vi "copy.vi"(8 "error in (no error)":errorcluster, 10 "ScriptEventForCopy":refnum<class "ScriptEvent.lvclass">, 11 "SingleToneRamp in":refnum<class "SingleToneRamp.lvclass">) -> (0 "error out":errorcluster, 3 "SingleToneRamp Copy":refnum<class "SingleToneRamp.lvclass">)   [LabVIEW 2011, in "Tools.lvlib" / "Scripting.lvlib" / "SingleToneRamp.lvclass"]
uses:
  SingleToneRamp.lvclass
  ScriptEvent.lvclass
  SingleTone.lvclass
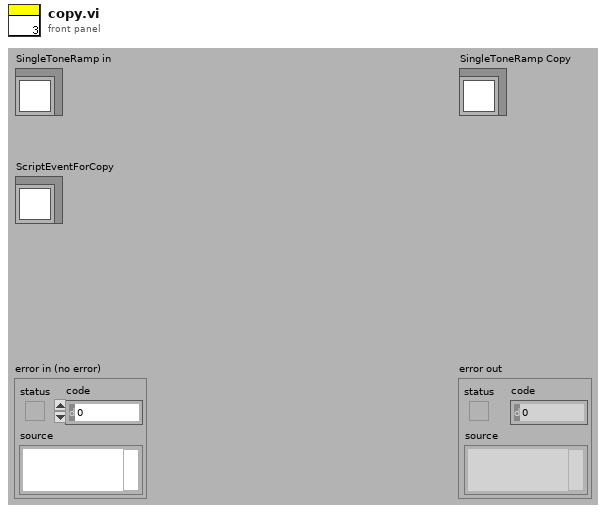
[diagram p1: front panel]
types:
  T1 = enum16{"changeValue", "pulse", "clock", "rampUp", "rampDown", "singleTone", "singleToneRamp", "playFile", "rf", "rfRamp", "delay"}
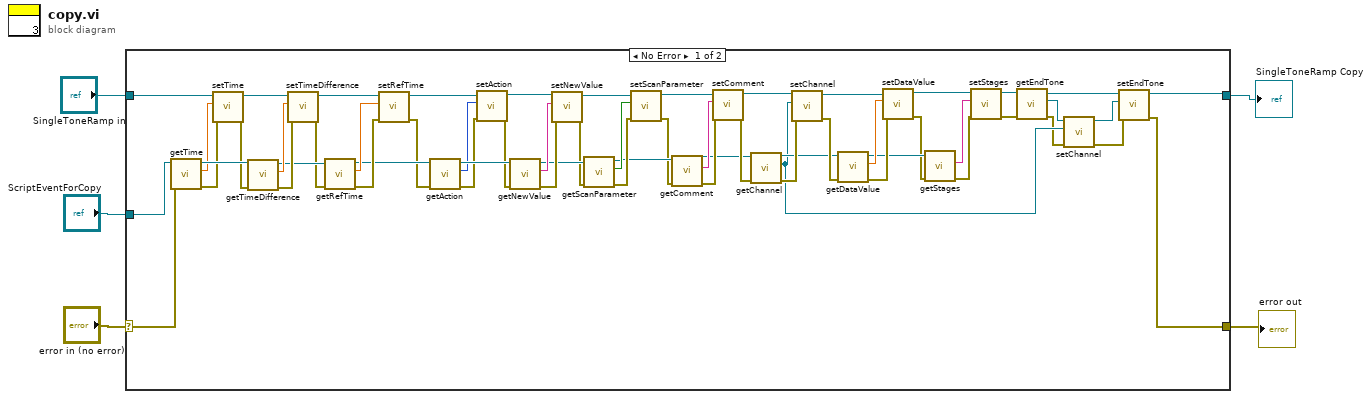
[diagram p0: block diagram]
diagram:
  n1 = case shown="No Error" "error in (no error)" {
    selector: "error in (no error)" -> [w15 w65]
    tunnel: "SingleToneRamp in" -> [w17 w66]
    tunnel: [w7 w66] -> w4
    tunnel: [w6 w65] -> w2
    tunnel: "ScriptEventForCopy" -> [w16 _]
    frame No Error {
      n2 = call "getTime.vi"("error in (no error)"=w15, "ScriptEvent.lvclass in"=w16) -> ("error out"=w63:errorcluster, "time"=w62:dbl, "ScriptEvent.lvclass out"=w64:refnum<class "ScriptEvent.lvclass">)  [unwired: 7 in]
      n3 = call "setTime.vi"("error in (no error)"=w63, "time"=w62, "ScriptEvent.lvclass in"=w17) -> ("error out"=w61:errorcluster, "ScriptEvent.lvclass out"=w33:refnum<class "SingleToneRamp.lvclass">)  [unwired: 7 in]
      n4 = call "getTimeDifference.vi"("error in (no error)"=w61, "ScriptEvent.lvclass in"=w64) -> ("error out"=w60:errorcluster, "time difference"=w34:dbl, "ScriptEvent.lvclass out"=w23:refnum<class "ScriptEvent.lvclass">)  [unwired: 7 in]
      n5 = call "setTimeDifference.vi"("error in (no error)"=w60, "time difference"=w34, "ScriptEvent.lvclass in"=w33) -> ("error out"=w22:errorcluster, "ScriptEvent.lvclass out"=w24:refnum<class "SingleToneRamp.lvclass">)  [unwired: 7 in]
      n6 = call "getRefTime.vi"("error in (no error)"=w22, "ScriptEvent.lvclass in"=w23) -> ("error out"=w20:errorcluster, "refTime"=w21:dbl, "ScriptEvent.lvclass out"=w19:refnum<class "ScriptEvent.lvclass">)  [unwired: 7 in]
      n7 = call "setRefTime.vi"("error in (no error)"=w20, "refTime"=w21, "ScriptEvent.lvclass in"=w24) -> ("error out"=w18:errorcluster, "ScriptEvent.lvclass out"=w25:refnum<class "SingleToneRamp.lvclass">)  [unwired: 7 in]
      n8 = call "getAction.vi"("error in (no error)"=w18, "ScriptEvent.lvclass in"=w19) -> ("error out"=w58:errorcluster, "action"=w57:T1, "ScriptEvent.lvclass out"=w59:refnum<class "ScriptEvent.lvclass">)  [unwired: 7 in]
      n9 = call "setAction.vi"("error in (no error)"=w58, "action"=w57, "ScriptEvent.lvclass in"=w25) -> ("error out"=w56:errorcluster, "ScriptEvent.lvclass out"=w32:refnum<class "SingleToneRamp.lvclass">)  [unwired: 7 in]
      n10 = call "getNewValue.vi"("error in (no error)"=w56, "ScriptEvent.lvclass in"=w59) -> ("error out"=w55:errorcluster, "newValue"=w54:string, "ScriptEvent.lvclass out"=w53:refnum<class "ScriptEvent.lvclass">)  [unwired: 7 in]
      n11 = call "setNewValue.vi"("error in (no error)"=w55, "newValue"=w54, "ScriptEvent.lvclass in"=w32) -> ("error out"=w52:errorcluster, "ScriptEvent.lvclass out"=w31:refnum<class "SingleToneRamp.lvclass">)  [unwired: 7 in]
      n12 = call "getScanParameter.vi"("error in (no error)"=w52, "ScriptEvent.lvclass in"=w53) -> ("error out"=w50:errorcluster, "scanParameter"=w51:bool, "ScriptEvent.lvclass out"=w49:refnum<class "ScriptEvent.lvclass">)  [unwired: 7 in]
      n13 = call "setScanParameter.vi"("error in (no error)"=w50, "scanParameter"=w51, "ScriptEvent.lvclass in"=w31) -> ("error out"=w48:errorcluster, "ScriptEvent.lvclass out"=w30:refnum<class "SingleToneRamp.lvclass">)  [unwired: 7 in]
      n14 = call "getComment.vi"("error in (no error)"=w48, "ScriptEvent.lvclass in"=w49) -> ("error out"=w47:errorcluster, "comment"=w46:string, "ScriptEvent.lvclass out"=w44:refnum<class "ScriptEvent.lvclass">)  [unwired: 7 in]
      n15 = call-dynamic "setComment.vi"("error in (no error)"=w47, "comment"=w46, "SingleToneRamp.lvclass in"=w30) -> ("error out"=w45:errorcluster, "SingleToneRamp.lvclass out"=w29:refnum<class "SingleToneRamp.lvclass">)  [unwired: 7 in]
      n16 = call-dynamic "getChannel.vi"("error in (no error)"=w45, "ScriptEvent.lvclass in"=w44) -> ("error out"=w43:errorcluster, "Channel.lvclass"=w26:refnum<class "Channel.lvclass">, "ScriptEvent.lvclass out"=w41:refnum<class "ScriptEvent.lvclass">)  [unwired: 7 in]
      n17 = call-dynamic "setChannel.vi"("error in (no error)"=w43, "Channel.lvclass"=w26, "SingleToneRamp.lvclass in"=w29) -> ("error out"=w42:errorcluster, "SingleToneRamp.lvclass out"=w28:refnum<class "SingleToneRamp.lvclass">)  [unwired: 7 in]
      n18 = call "getDataValue.vi"("error in (no error)"=w42, "ScriptEvent.lvclass in"=w41) -> ("error out"=w40:errorcluster, "dataValue"=w39:dbl, "ScriptEvent.lvclass out"=w38:refnum<class "ScriptEvent.lvclass">)  [unwired: 7 in]
      n19 = call "setDataValue.vi"("error in (no error)"=w40, "dataValue"=w39, "ScriptEvent.lvclass in"=w28) -> ("error out"=w37:errorcluster, "ScriptEvent.lvclass out"=w27:refnum<class "SingleToneRamp.lvclass">)  [unwired: 7 in]
      n20 = call "getStages.vi"("error in (no error)"=w37, "ScriptEvent.lvclass in"=w38) -> ("error out"=w36:errorcluster, "Stage"=w35:string)  [unwired: 7 in, 1 out]
      n21 = call-dynamic "setStages.vi"("error in (no error)"=w36, "Stage"=w35, "SingleToneRamp.lvclass in"=w27) -> ("error out"=w10:errorcluster, "SingleToneRamp.lvclass out"=w14:refnum<class "SingleToneRamp.lvclass">)  [unwired: 7 in]
      n22 = call "getEndTone.vi"("error in (no error)"=w10, "SingleToneRamp.lvclass in"=w14) -> ("error out"=w11:errorcluster, "endTone"=w12:refnum<class "SingleTone.lvclass">, "SingleToneRamp.lvclass out"=w13:refnum<class "SingleToneRamp.lvclass">)  [unwired: 7 in]
      n23 = call-dynamic "setChannel.vi"("error in (no error)"=w11, "Channel.lvclass"=w26, "ScriptEvent.lvclass in"=w12) -> ("error out"=w8:errorcluster, "ScriptEvent.lvclass out"=w9:refnum<class "SingleTone.lvclass">)  [unwired: 7 in]
      n24 = call "setEndTone.vi"("error in (no error)"=w8, "EndTone"=w9, "SingleToneRamp.lvclass in"=w13) -> ("error out"=w6:errorcluster, "SingleToneRamp.lvclass out"=w7:refnum<class "SingleToneRamp.lvclass">)  [unwired: 7 in]
    }
    frame Error {
    }
  }
  "error out" <- w2
  "SingleToneRamp Copy" <- w4
